vi "ShowLineColor.vi"(8 "ColorIn":u32, 9 "TestingIndex":i32, 10 "color":T1(ring), 11 "MulticolumnListbox in":refnum<vi>) -> ()   [LabVIEW 2018]
uses:
  <vilib>/Utility/miscctls.llb/LVRowAndColumnTypeDef.ctl
panel:
  out "error out":errorcluster
  out "reference out":refnum<vi>
  in  "error in (no error)":errorcluster
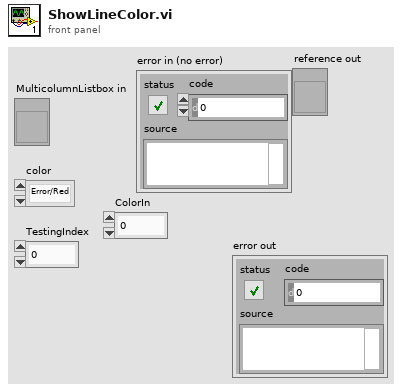
[diagram p1: front panel]
types:
  T1 = enum16{"Error/Red", "Null/White", "OK/Green", "Warnnig/Yellow", "Testing/SkyBlue"}
  T2 = typedef "LVRowAndColumnTypeDef.ctl" = cluster{"Row":i32, "Column":i32}
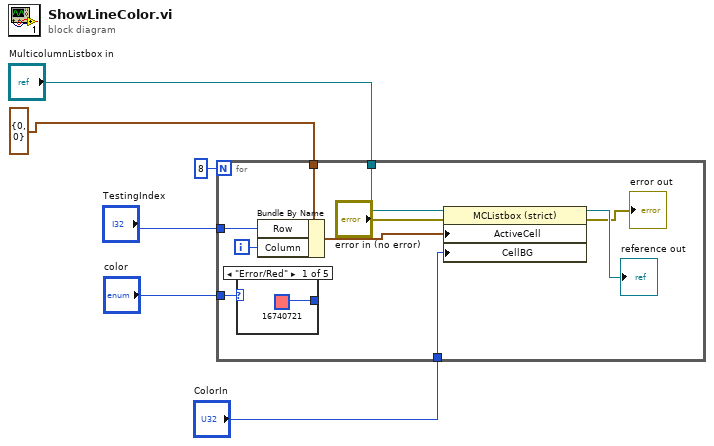
[diagram p0: block diagram]
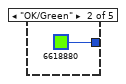
[diagram p2: hidden frame]
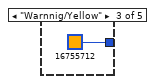
[diagram p3: hidden frame]
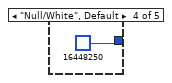
[diagram p4: hidden frame]
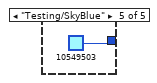
[diagram p5: hidden frame]
diagram:
  n1 = for {
    N: 8 -> [_]
    tunnel: "color" -> [w16]
    tunnel: "TestingIndex" -> [w14]
    tunnel: T2 {"Row"=0, "Column"=0} ("Active Cell:Active Cell") -> [w13]
    tunnel: "MulticolumnListbox in" -> [w12]
    tunnel: "ColorIn" -> [w7]
    i -> [w11]
    n2 = case shown="\"Error/Red\"" w16 {
      tunnel: [u32 16740721 u32 6618880 u32 16755712 u32 16448250 u32 10549503] -> _
      frame "Error/Red" {
      }
      frame "OK/Green" {
      }
      frame "Warnnig/Yellow" {
      }
      frame "Null/White", Default {
      }
      frame "Testing/SkyBlue" {
      }
    }
    n3 = Bundle By Name(cluster=w13, "Row"=w14, "Column"=w11) -> (w15:T2)
    n4 = property on="Property Node" class="MCListbox (strict)"(reference=w12, error in="error in (no error)", "ActiveCell"=w15, "CellBG"=w7) -> (reference out=→"reference out":refnum<vi>, error out=→"error out":errorcluster)
  }
